vi "GetFaultListBatt_module.vi"(1 "Module Number":i32, 2 "Warn":u16 format="%x", 3 "Err1":u16 format="%x") -> (0 "Error/Warning":string)   [LabVIEW 2021]
panel:
  in  "Warn string":string[](array[string])=["", "Reduced power to prevent overvoltage", "Reduced power to prevent undervoltage", "Reduced power due to undertemperature", "Reduced power due to overertemperature", "", "", "", "", "Yellow flag", "Watchdog disabled", "", "", "", "", ""]
  in  "Err1 string":string[](array[string])=["OverCurrent", "OvervVoltage", "UnderVoltage", "UnderTemperature", "OverTemperature", "SelfTest Error", "DC-power cable missing", "External stop from I/O", "Incompatible SRB modules in string", "Fan error (SRB)", "Broken wire detected", "Communication error current sensor", "Communication error second level safety", "Thirs level safety error", "Contactor error", "Service Necessary"]
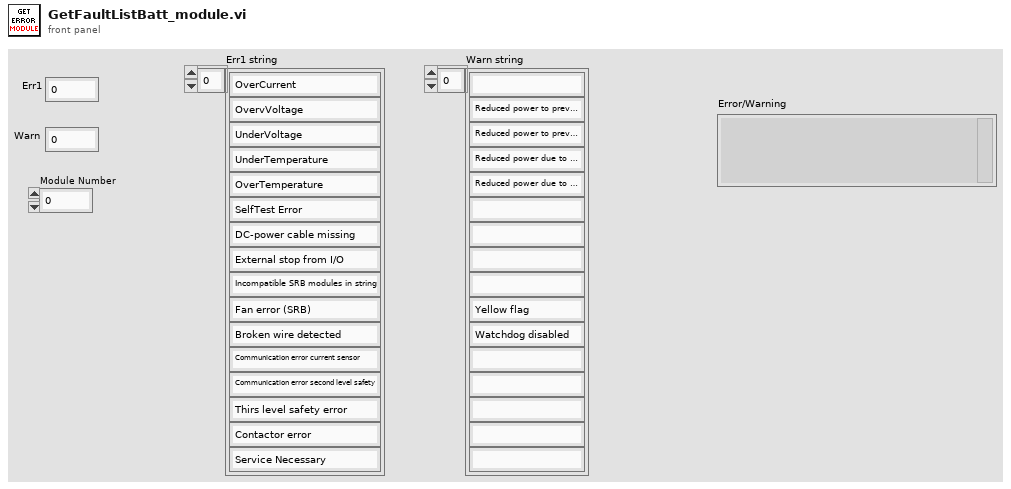
[diagram p1: front panel]
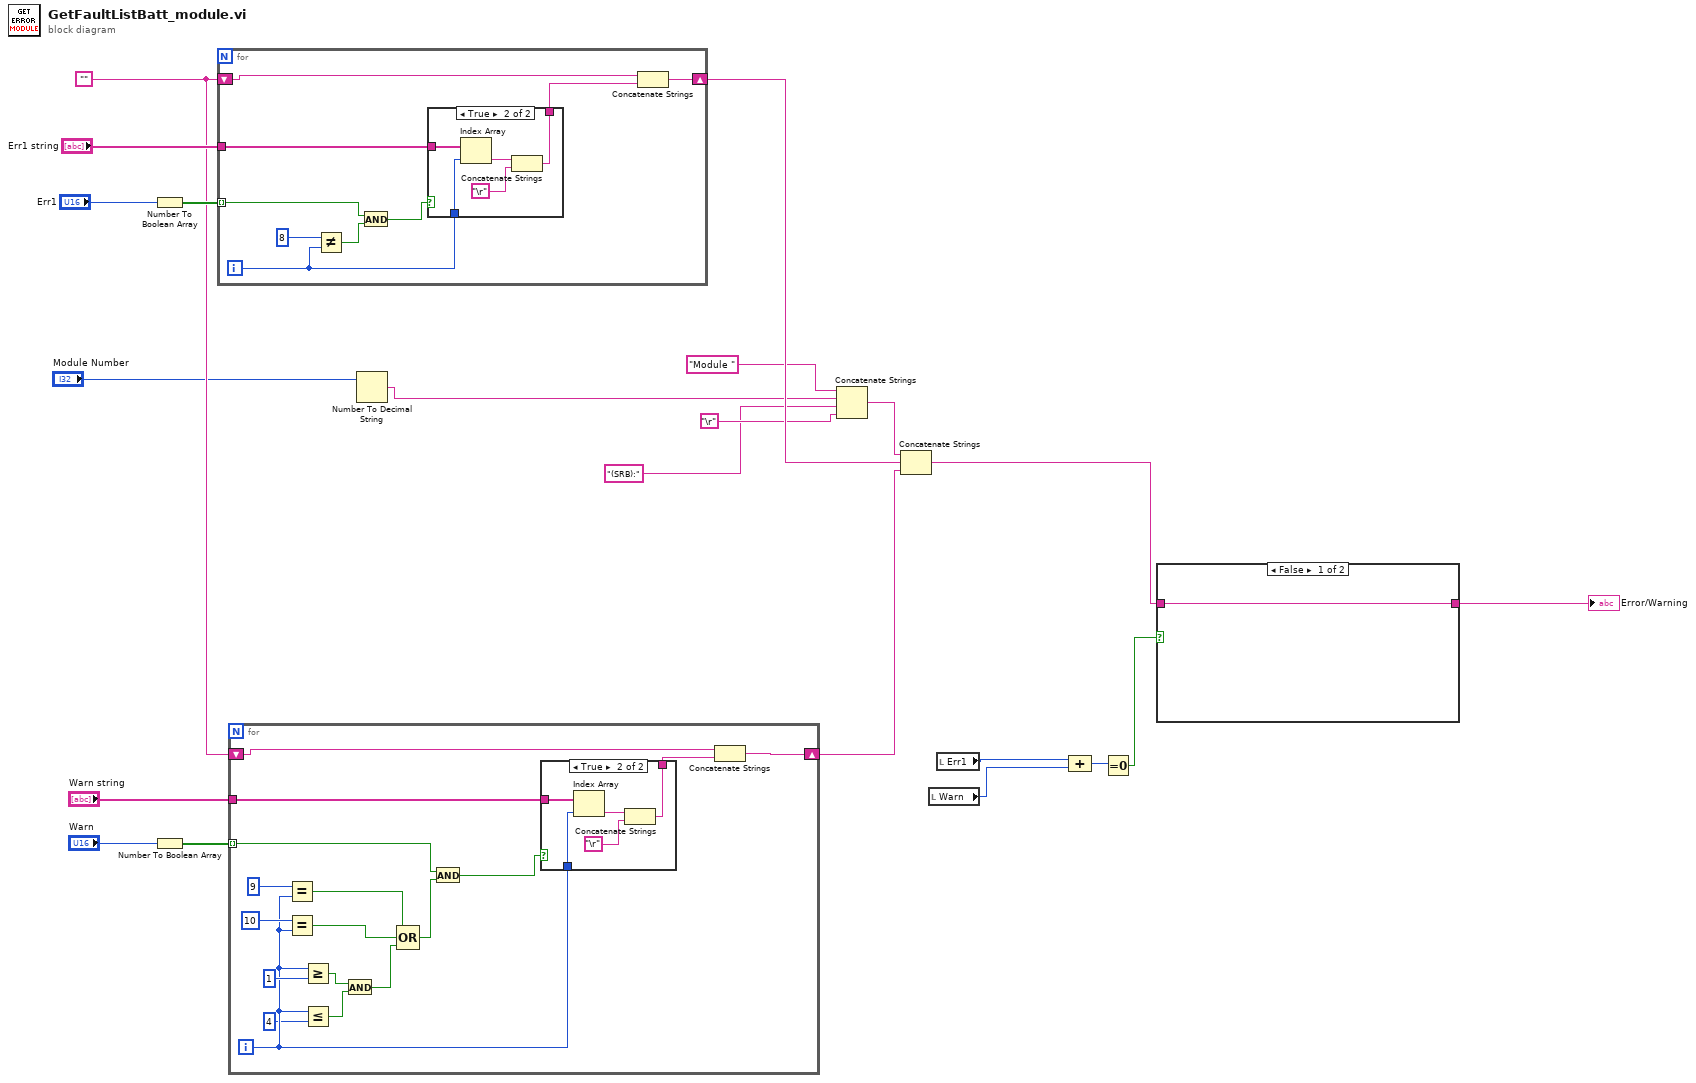
[diagram p0: block diagram]
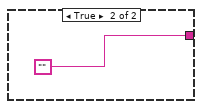
[diagram p2: hidden frame]
diagram:
  w15 = ""
  n1 = Number To Boolean Array(number="Err1") -> (Boolean array=w19:bool[])
  n2 = Number To Boolean Array(number="Warn") -> (Boolean array=w12:bool[])
  n3 = for {
    tunnel: "Err1 string" -> [w30]
    tunnel: w19 -> [w23] mode=indexing
    shift-right: [w28] -> w18
    shift-left: w15 -> [w29]
    i -> [w26]
    n4 = Not Equal?(x=8, y=w26) -> (x != y?=w24:bool)
    n5 = And(x=w23, y=w24) -> (x .and. y?=w22:bool)
    n6 = case shown="True" w22 {
      tunnel: w30 -> [_ w32]
      tunnel: w26 -> [_ w35]
      tunnel: [_ w33] -> w27
      frame False {
      }
      frame True {
        n7 = Index Array(array=w32, index=w35) -> (element=w31:string)
        n8 = Concatenate Strings(w31, "\r") -> (w33:string)
      }
    }
    n9 = Concatenate Strings(w29, w27) -> (w28:string)
  }
  n10 = for {
    shift-right: [w51] -> w11
    shift-left: w15 -> [w52]
    tunnel: "Warn string" -> [w48]
    tunnel: w12 -> [w43] mode=indexing
    i -> [w40]
    n11 = Equal?(x=9, y=w40) -> (x = y?=w45:bool)
    n12 = Equal?(x=10, y=w40) -> (x = y?=w46:bool)
    n13 = Greater Or Equal?(x=w40, y=1) -> (x >= y?=w38:bool)
    n14 = Less Or Equal?(x=w40, y=4) -> (x <= y?=w37:bool)
    n15 = And(x=w38, y=w37) -> (x .and. y?=w36:bool)
    n16 = Compound Arithmetic op=OR(w45, w46, w36) -> (w42:bool)
    n17 = And(x=w43, y=w42) -> (x .and. y?=w44:bool)
    n18 = case shown="True" w44 {
      tunnel: w48 -> [_ w54]
      tunnel: w40 -> [_ w57]
      tunnel: [_ w55] -> w50
      frame False {
      }
      frame True {
        n19 = Index Array(array=w54, index=w57) -> (element=w53:string)
        n20 = Concatenate Strings(w53, "\r") -> (w55:string)
      }
    }
    n21 = Concatenate Strings(w52, w50) -> (w51:string)
  }
  n22 = Number To Decimal String(number="Module Number") -> (decimal integer string=w6:string)  [unwired: 1 in]
  n23 = Concatenate Strings("Module " ("string"), w6, "(SRB):" ("string"), "\r") -> (w16:string)
  n24 = Concatenate Strings(w16, w18, w11) -> (w3:string)
  n25 = local read "Warn"() -> (w1:u16)
  n26 = local read "Err1"() -> (w2:u16)
  n27 = Compound Arithmetic op=ADD(w2, w1) -> (w10:u16)
  n28 = Equal To 0?(x=w10) -> (x = 0?=w9:bool)
  n29 = case shown="False" w9 {
    tunnel: [w58 ""] -> w8
    tunnel: w3 -> [w58 _]
    frame False {
    }
    frame True {
    }
  }
  "Error/Warning" <- w8
